vi "Configure Frequency.vi"(0 "VISA resource name":refnum<visa-resource-name>, 1 "Resolution (7: 7 digits)":u16(ring)=7 items=["4 Digits"=4, "5 Digits"=5, "6 Digits"=6, "7 Digits"=7], 5 "error in (no error)":errorcluster, 8 "Threshold Range (10 V)":dbl=10.0 format="%#_6p", 10 "Reference (0: Off)":u16(ring) items=["Off", "Set", "Acquire"], 12 "Reference Value (0.000 Hz)":dbl format="%_3g") -> (14 "VISA resource name out":refnum<visa-resource-name>, 19 "error out":errorcluster)   [LabVIEW 2020, in "Keithley 2000.lvlib"]
doc: "This VI configures the instrument to measure the frequency of an AC signal."
uses:
  <instrlib>/Keithley 2000/Keithley 2000.lvlib
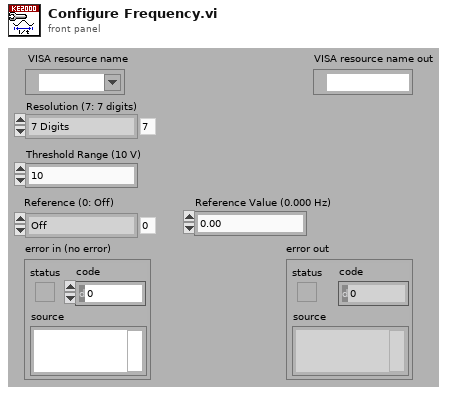
[diagram p1: front panel]
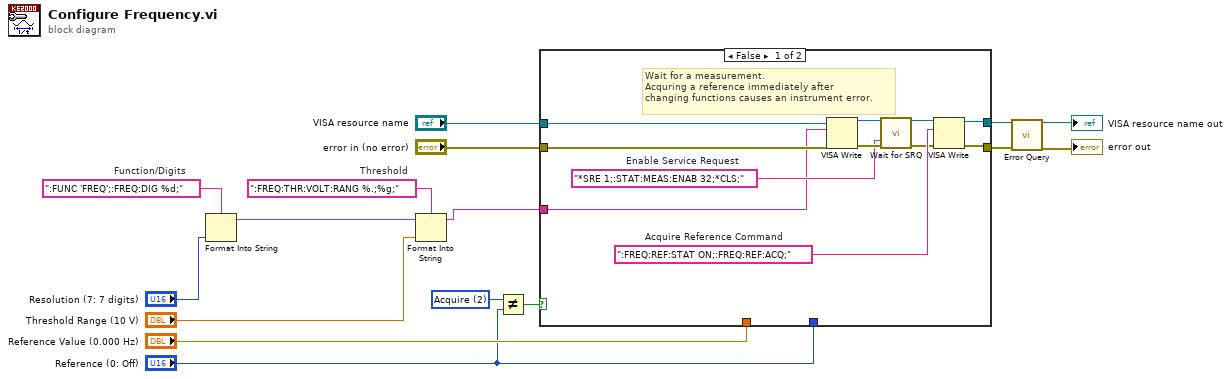
[diagram p0: block diagram]
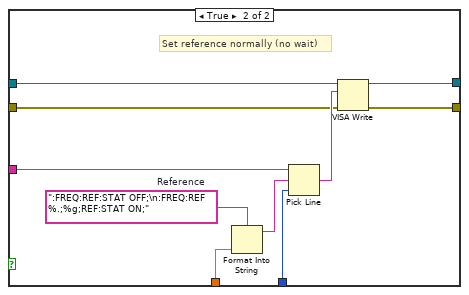
[diagram p2: hidden frame]
diagram:
  w9 = u16 2 items=["Off", "Set", "Acquire"] ("Reference (0: Off)")
  w14 = ":FREQ:THR:VOLT:RANG %.;%g;"  # Threshold
  w15 = ":FUNC 'FREQ';:FREQ:DIG %d;"  # Function/Digits
  n1 = Format Into String(format string=w15, "Resolution (7: 7 digits)") -> (resulting string=w12:string)  [unwired: 2 in, 1 out]
  n2 = Format Into String(format string=w14, initial string=w12, "Threshold Range (10 V)") -> (resulting string=w1:string)  [unwired: 1 in, 1 out]
  n3 = Not Equal?(x=w9, y="Reference (0: Off)") -> (x != y?=w3:bool)
  n4 = case shown="False" w3 {
    tunnel: "VISA resource name" -> [w24 w30]
    tunnel: "error in (no error)" -> [w25 w29]
    tunnel: "Reference Value (0.000 Hz)" -> [_ w35]
    tunnel: w1 -> [w17 w28]
    tunnel: [w19 w34] -> w5
    tunnel: [w20 w33] -> w6
    tunnel: "Reference (0: Off)" -> [_ w31]
    frame False {
      w18 = "*SRE 1;:STAT:MEAS:ENAB 32;*CLS;"  # Enable Service Request
      w23 = ":FREQ:REF:STAT ON;:FREQ:REF:ACQ;"  # Acquire Reference Command
      # "Wait for a measurement.\nAcquring a reference immediately after\nchanging functions causes an instrument error."
      n5 = VISA Write(VISA resource name=w24, write buffer=w17, error in (no error)=w25) -> (VISA resource name out=w27:refnum<visa-resource-name>, error out=w26:errorcluster)  [unwired: 1 out]
      n6 = call <instrlib>:"Wait for SRQ.vi"("VISA resource name"=w27, "SRQ Enable Command"=w18, "error in (no error)"=w26) -> ("VISA resource name out"=w22:refnum<visa-resource-name>, "error out"=w21:errorcluster)  [unwired: 15 in]
      n7 = VISA Write(VISA resource name=w22, write buffer=w23, error in (no error)=w21) -> (VISA resource name out=w20:refnum<visa-resource-name>, error out=w19:errorcluster)  [unwired: 1 out]
    }
    frame True {
      w37 = ":FREQ:REF:STAT OFF;\n:FREQ:REF %.;%g;REF:STAT ON;"  # Reference
      # "Set reference normally (no wait)"
      n8 = Format Into String(format string=w37, w35) -> (resulting string=w36:string)  [unwired: 2 in, 1 out]
      n9 = Pick Line(string ("")=w28, multi-line string=w36, line index=w31) -> (output string=w32:string)
      n10 = VISA Write(VISA resource name=w30, write buffer=w32, error in (no error)=w29) -> (VISA resource name out=w33:refnum<visa-resource-name>, error out=w34:errorcluster)  [unwired: 1 out]
    }
  }
  n11 = call <instrlib>:"Error Query.vi"("VISA resource name"=w6, "error in (no error)"=w5) -> ("VISA resource name out"=→"VISA resource name out":refnum<visa-resource-name>, "error out"=→"error out":errorcluster)  [unwired: 14 in, 2 out]
